vi "ParceCFG.vi"(1 "path":path) -> ()   [LabVIEW 2010]
panel:
  out "Valid":bool
  out "VM DESCR":T1
  out "VP DESCR":T2
  out "CA DESCR":T3
  out "CA_COM2AY":T4(array[cluster])
  out "CA_AY2GUI":T4(array[cluster])
  out "VOC Cluster Array":T4(array[cluster])
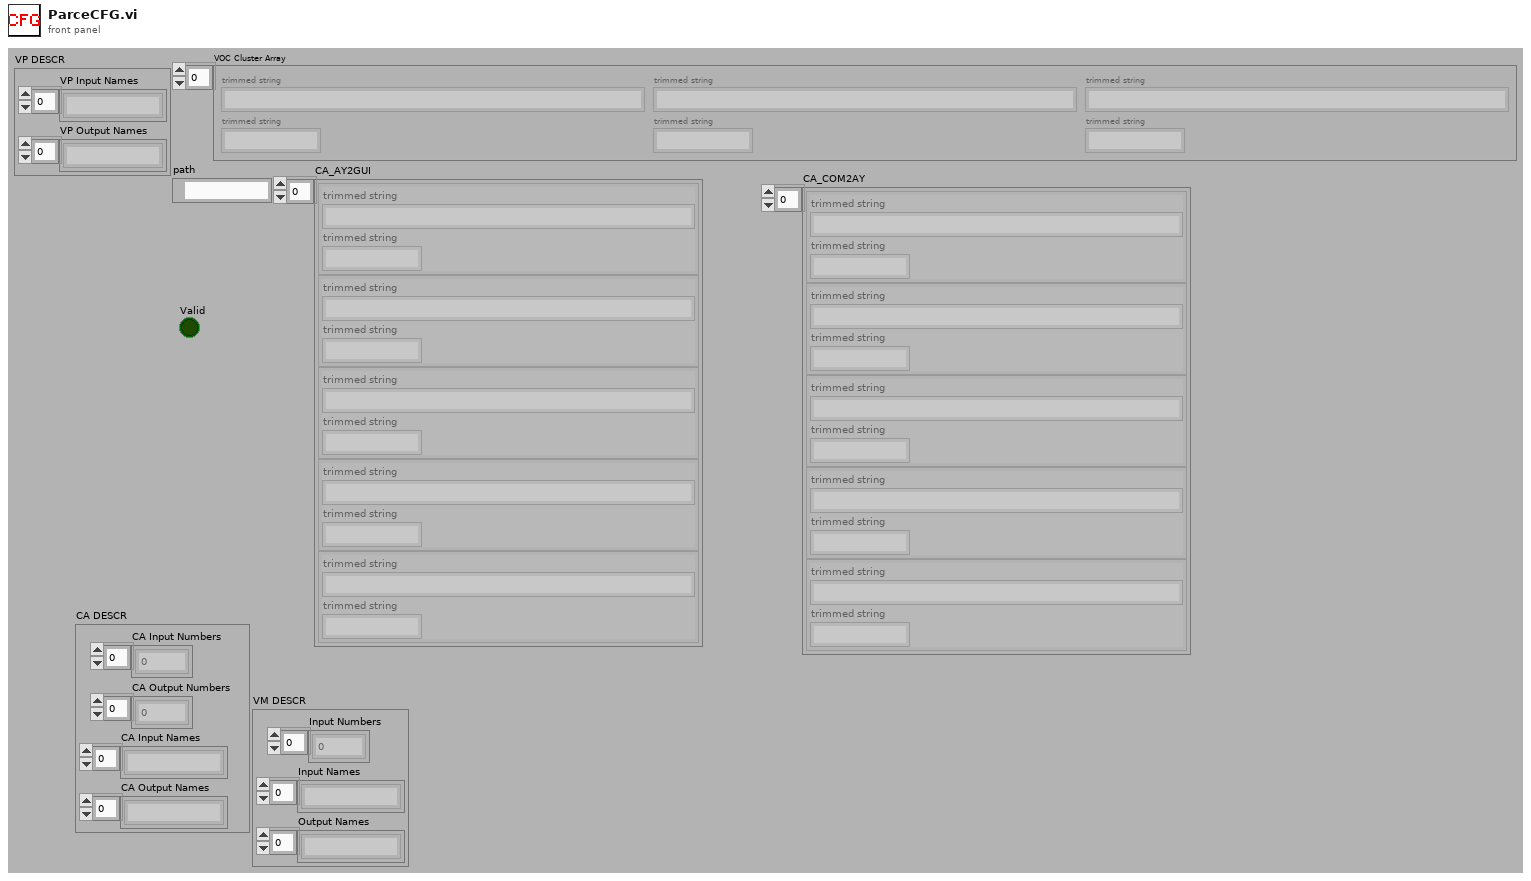
[diagram p1: front panel]
types:
  T1 = cluster{"Input Numbers":i32[], "Input Names":string[], "Output Names ":string[]}
  T2 = cluster{"VP Input Names":string[], "VP Output Names ":string[]}
  T3 = cluster{"CA Input Numbers":i32[], "CA Output Numbers ":i32[], "CA Input Names":string[], "CA Output Names ":string[]}
  T4 = cluster{"trimmed string":string, "trimmed string":string}[]
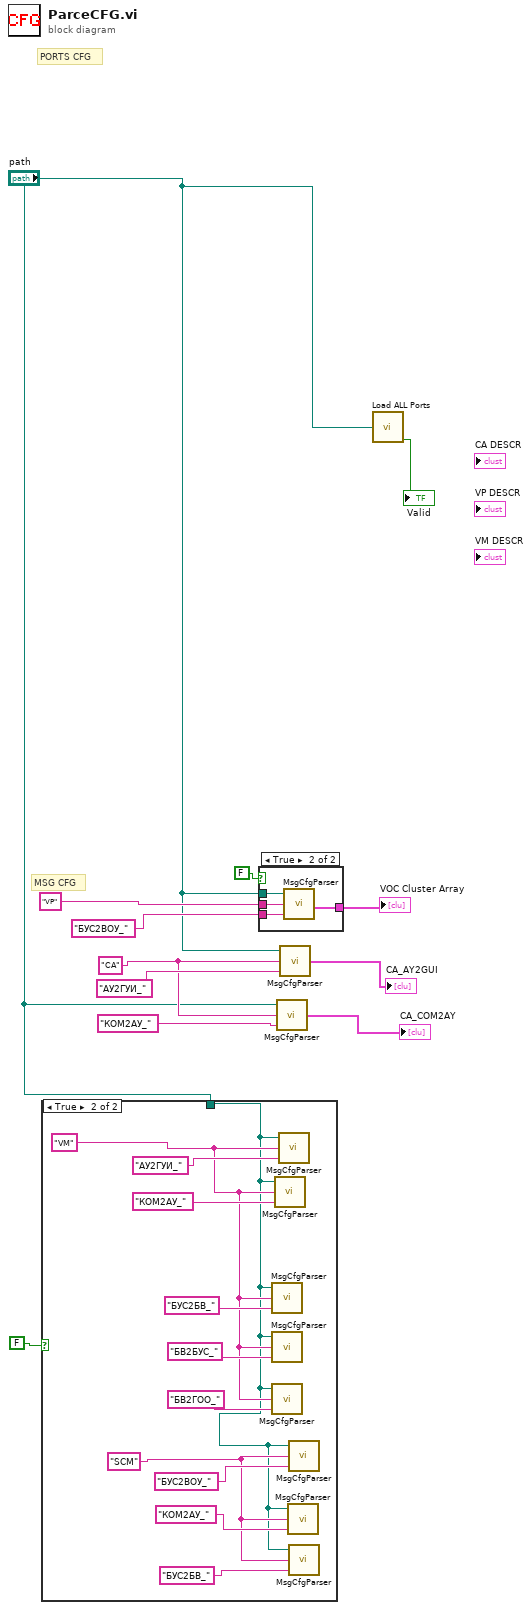
[diagram p0: block diagram]
diagram:
  w8 = "CA" ("name or relative path")
  # "MSG CFG"
  # "PORTS CFG"
  n1 = case shown="True" FALSE {
    tunnel: "path" -> [_ w13]
    frame False {
    }
    frame True {
      w14 = "SCM" ("name or relative path")
      w18 = "VM" ("name or relative path")
      n2 = call "MsgCfgParser.vi"("search string"="БУС2БВ_" ("name or relative path"), "name or relative path"=w18, "stripped path"=w13) -> ()  [unwired: 1 out]
      n3 = call "MsgCfgParser.vi"("search string"="БВ2БУС_" ("name or relative path"), "name or relative path"=w18, "stripped path"=w13) -> ()  [unwired: 1 out]
      n4 = call "MsgCfgParser.vi"("search string"="БВ2ГОО_" ("name or relative path"), "name or relative path"=w18, "stripped path"=w13) -> ()  [unwired: 1 out]
      n5 = call "MsgCfgParser.vi"("search string"="КОМ2АУ_" ("name or relative path"), "name or relative path"=w18, "stripped path"=w13) -> ()  [unwired: 1 out]
      n6 = call "MsgCfgParser.vi"("search string"="АУ2ГУИ_" ("name or relative path"), "name or relative path"=w18, "stripped path"=w13) -> ()  [unwired: 1 out]
      n7 = call "MsgCfgParser.vi"("search string"="КОМ2АУ_" ("name or relative path"), "name or relative path"=w14, "stripped path"=w13) -> ()  [unwired: 1 out]
      n8 = call "MsgCfgParser.vi"("search string"="БУС2ВОУ_" ("name or relative path"), "name or relative path"=w14, "stripped path"=w13) -> ()  [unwired: 1 out]
      n9 = call "MsgCfgParser.vi"("search string"="БУС2БВ_" ("name or relative path"), "name or relative path"=w14, "stripped path"=w13) -> ()  [unwired: 1 out]
    }
  }
  n10 = case shown="True" FALSE {
    tunnel: "VP" ("name or relative path") -> [_ w27]
    tunnel: [_ w26] -> w11
    tunnel: "БУС2ВОУ_" ("name or relative path") -> [_ w25]
    tunnel: "path" -> [_ w24]
    frame False {
    }
    frame True {
      n11 = call "MsgCfgParser.vi"("search string"=w25, "name or relative path"=w27, "stripped path"=w24) -> ("Cluster Array"=w26:T4)
    }
  }
  "VOC Cluster Array" <- w11
  n12 = call "MsgCfgParser.vi"("search string"="КОМ2АУ_" ("name or relative path"), "name or relative path"=w8, "stripped path"="path") -> ("Cluster Array"=→"CA_COM2AY":T4)
  n13 = call "MsgCfgParser.vi"("search string"="АУ2ГУИ_" ("name or relative path"), "name or relative path"=w8, "stripped path"="path") -> ("Cluster Array"=→"CA_AY2GUI":T4)
  n14 = call "Load ALL Ports.vi"("path"="path") -> ("VALID"=→"Valid":bool)  [unwired: 3 out]
